vi "TCP IP Parse BipolarMode.vi"(11 "JSON in":string) -> (2 "Value":T1, 3 "JSON out":string)   [LabVIEW 2015]
uses:
  Controls/Control_Fornax Bipolar Enum.ctl
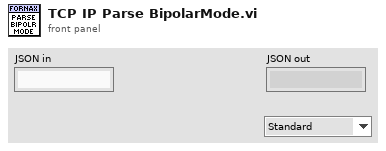
[diagram p1: front panel]
types:
  T1 = typedef "Control_Fornax Bipolar Enum.ctl" = enum16{"Standard", "Macro", "Precision"}
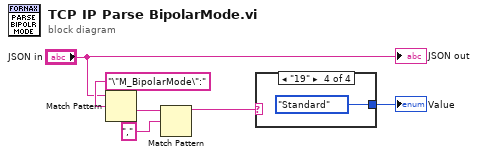
[diagram p0: block diagram]
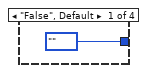
[diagram p2: hidden frame]
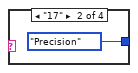
[diagram p3: hidden frame]
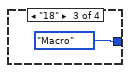
[diagram p4: hidden frame]
diagram:
  n1 = Match Pattern(string="JSON in", regular expression="\"M_BipolarMode\":") -> (after substring=w4:string)  [unwired: 1 in, 3 out]
  n2 = Match Pattern(string=w4, regular expression=",") -> (before substring=w6:string)  [unwired: 1 in, 3 out]
  n3 = case shown="\"19\"" w6 {
    tunnel: [enum16{""}."" Control_Fornax_Bipolar_Enum."Precision" ("Value") Control_Fornax_Bipolar_Enum."Macro" ("Value") Control_Fornax_Bipolar_Enum."Standard" ("Value")] -> w1
    frame "False", Default {
    }
    frame "17" {
    }
    frame "18" {
    }
    frame "19" {
    }
  }
  "Value" <- w1
  "JSON out" <- "JSON in"
